vi "flip_2D_I32_array_td.vi"(1 "Half Centerline Pixel Sequence":i32[][](array[numeric])) -> (0 "Array Flipped Top Down":i32[][](array[numeric]))   [LabVIEW 2019]
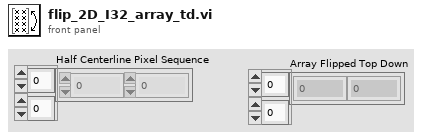
[diagram p1: front panel]
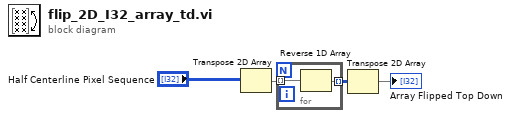
[diagram p0: block diagram]
diagram:
  n1 = Transpose 2D Array(2D array="Half Centerline Pixel Sequence") -> (transposed array=w4:i32[][])
  n2 = for {
    tunnel: w4 -> [w6] mode=indexing
    tunnel: [w5] -> w3 mode=indexing
    n3 = Reverse 1D Array(array=w6) -> (reversed array=w5:i32[])
  }
  n4 = Transpose 2D Array(2D array=w3) -> (transposed array=→"Array Flipped Top Down":i32[][])
